vi "Send Template.vi"(4 "TimeOut":dbl[unit]=10.0 format="%#_13g", 6 "CallerParameter":cluster{}, 7 "Message Priority (Normal)":T1=enum."Normal", 8 "error in (no error)":errorcluster, 9 "AcknowledgeMsg":refnum<class "Message.lvclass">, 10 "Acknowledge Receiver":refnum<class "Message Enqueuer.lvclass">, 11 "Message Enqueuer":refnum<class "Message Enqueuer.lvclass">) -> (0 "error out":errorcluster, 3 "Message Enqueuer out":refnum<class "Message Enqueuer.lvclass">)   [LabVIEW 2016, in "AsynchReturnDialog Template.lvclass"]
doc: "This VI sends the message to an actor."
uses:
  AsynchReturnDialog Template.lvclass
  <vilib>/ActorFramework/Message Enqueuer/Message Enqueuer.lvclass
  <vilib>/ActorFramework/Message/Message.lvclass
  <vilib>/ActorFramework/Actor/Actor.lvclass
  <vilib>/ActorFramework/Message Enqueuer/Message Priority.ctl
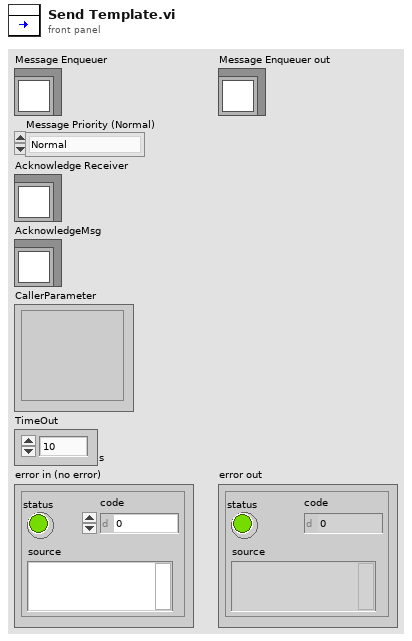
[diagram p1: front panel]
types:
  T1 = typedef "Actor Framework.lvlib/Message Enqueuer.lvclass/Message Priority.ctl" = enum16{"Low", "Normal", "High"}
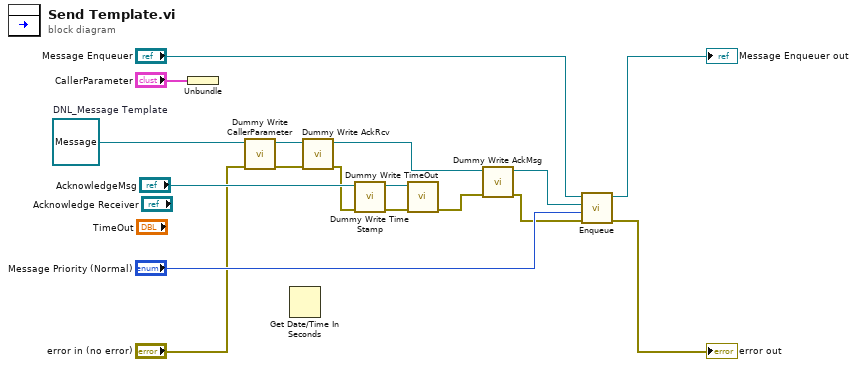
[diagram p0: block diagram]
diagram:
  w7 = refnum<class "Message.lvclass"> refnum  # DNL_Message Template
  n1 = Unbundle ("Unbundler")("CallerParameter") -> ()  [unwired: 1 out]
  n2 = call "Dummy Write CallerParameter.vi"("error in (no error)"="error in (no error)", "Actor in"=w7) -> ("error out"=w5:errorcluster, "Actor out"=w3:refnum<class "Actor.lvclass">)  [unwired: 7 in]
  n3 = Get Date/Time In Seconds() -> ()  [unwired: 1 out]
  n4 = call "Dummy Write AckRcv.vi"("error in (no error)"=w5, "Actor in"=w3) -> ("error out"=w4:errorcluster, "Actor out"=w2:refnum<class "Actor.lvclass">)  [unwired: 7 in]
  n5 = call "Dummy Write Time Stamp.vi"("error in (no error)"=w4, "Actor in"="AcknowledgeMsg") -> ("error out"=w11:errorcluster, "Actor out"=w12:refnum<class "Actor.lvclass">)  [unwired: 8 in]
  n6 = call "Dummy Write TimeOut.vi"("error in (no error)"=w11, "Actor in"=w12) -> ("error out"=w10:errorcluster)  [unwired: 7 in, 1 out]
  n7 = call "Dummy Write AckMsg.vi"("error in (no error)"=w10, "Actor in"=w2) -> ("error out"=w9:errorcluster, "Actor out"=w8:refnum<class "Actor.lvclass">)  [unwired: 8 in]
  n8 = call <vilib>:"Enqueue.vi"("error in (no error)"=w9, "Message Priority (Normal)"="Message Priority (Normal)", "Message"=w8, "Message Enqueuer in"="Message Enqueuer") -> ("error out"=→"error out":errorcluster, "Message Enqueuer out"=→"Message Enqueuer out":refnum<class "Message Enqueuer.lvclass">)  [unwired: 6 in]
